vi "Get All Routing Channel Ref IDs.vi"(8 "error in":errorcluster, 11 "routing channels in":T1 format="%.0x") -> (0 "error out":errorcluster, 2 "all routing channels":T1[](array[typedef]) format="%.0x", 3 "routing channels out":T1 format="%.0x")   [LabVIEW 2020, in "Routing and Faulting Scripting.lvlib"]
doc: "Returns all routing channels of a Routing and Faulting custom device."
uses:
  Routing and Faulting Scripting.lvlib
  <vilib>/NI VeriStand/Custom Device API/Custom Device Item Ref.ctl
  <vilib>/NI VeriStand/Custom Device Tools/Custom Device Utility Library/Custom Device Utility Library.lvlib
  <vilib>/NI VeriStand/Custom Device API/Custom Device API.lvlib
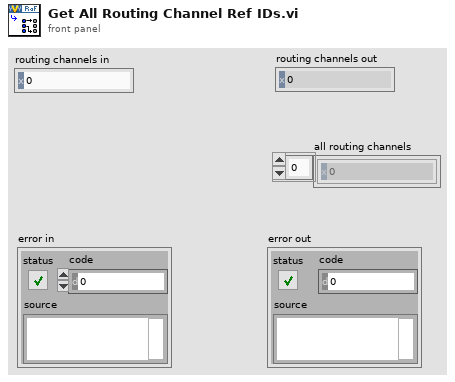
[diagram p1: front panel]
types:
  T1 = typedef "Custom Device API.lvlib/Custom Device Item Ref.ctl" = u64
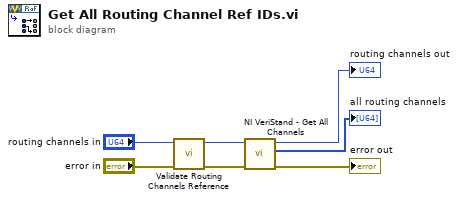
[diagram p0: block diagram]
diagram:
  n1 = call "Validate Routing Channels Reference.vi"("error in"="error in", "routing channels in"="routing channels in") -> ("error out"=w3:errorcluster, "routing channels out"=w1:T1)  [unwired: 8 in]
  n2 = call <vilib>:"NI VeriStand - Get All Channels.vi"("error in"=w3, "Section Ref in"=w1) -> ("error out"=→"error out":errorcluster, "Channel Refs"=→"all routing channels":T1[], "Section Ref out"=→"routing channels out":T1)  [unwired: 6 in, 1 out]
